vi "240913.vi"() -> ()   [LabVIEW 2024]
panel:
  in  "stop":bool
  in  "num":i8
  out "?":bool
  out "?":bool
  out "?":bool
  out "?":bool
  out "?":bool
  out "?":bool
  out "?":bool
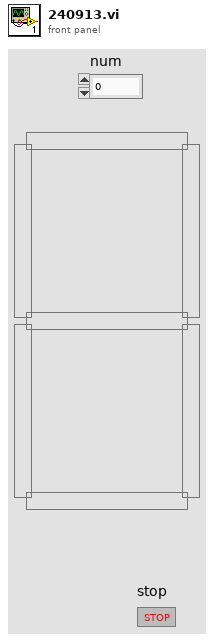
[diagram p1: front panel]
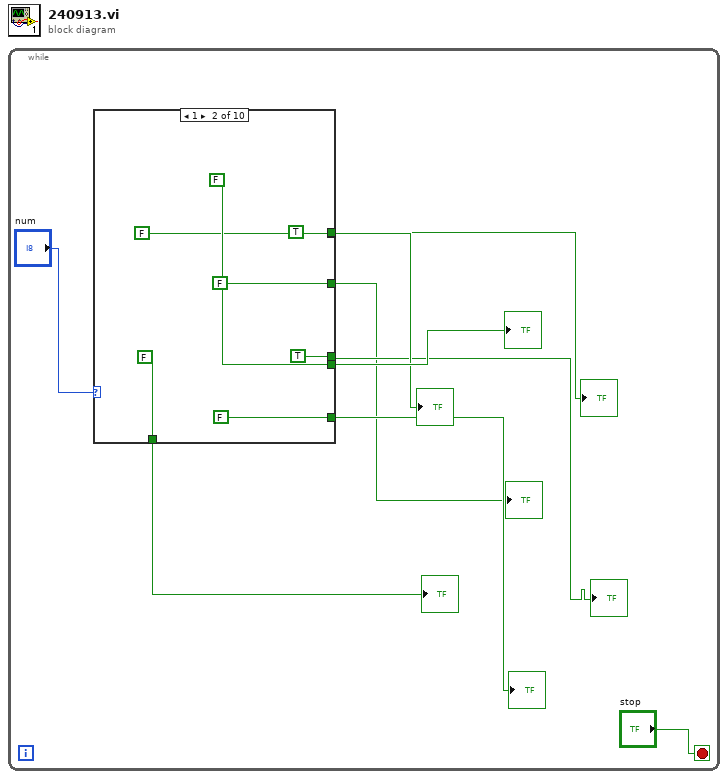
[diagram p0: block diagram]
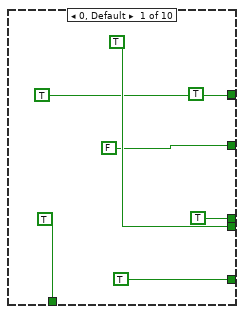
[diagram p2: hidden frame]
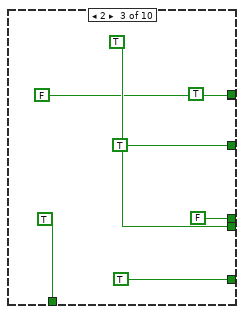
[diagram p3: hidden frame]
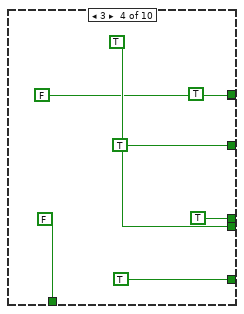
[diagram p4: hidden frame]
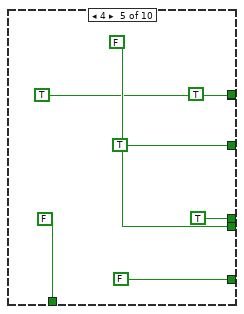
[diagram p5: hidden frame]
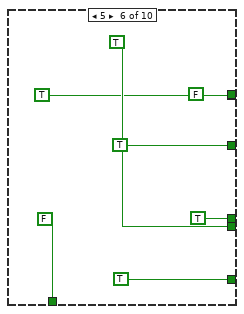
[diagram p6: hidden frame]
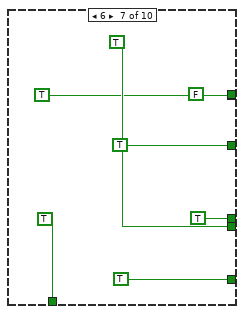
[diagram p7: hidden frame]
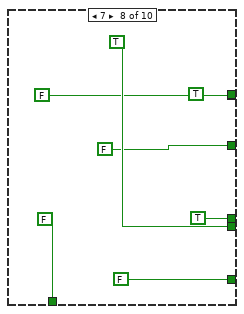
[diagram p8: hidden frame]
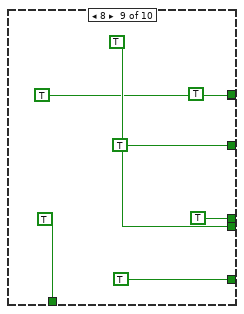
[diagram p9: hidden frame]
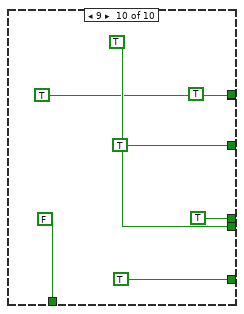
[diagram p10: hidden frame]
diagram:
  n1 = while {
    stop <- "stop" stop-if-true
    n2 = case shown="1" "num" {
      tunnel: [TRUE ("OK Button") FALSE ("OK Button") TRUE ("OK Button") TRUE ("OK Button") FALSE ("OK Button") TRUE ("OK Button") TRUE ("OK Button") TRUE ("OK Button") TRUE ("OK Button") TRUE ("OK Button")] -> w9
      tunnel: [TRUE ("OK Button") FALSE ("OK Button") FALSE ("OK Button") FALSE ("OK Button") TRUE ("OK Button") TRUE ("OK Button") TRUE ("OK Button") FALSE ("OK Button") TRUE ("OK Button") TRUE ("OK Button")] -> w8
      tunnel: [TRUE ("OK Button") FALSE ("OK Button") TRUE ("OK Button") FALSE ("OK Button") FALSE ("OK Button") FALSE ("OK Button") TRUE ("OK Button") FALSE ("OK Button") TRUE ("OK Button") FALSE ("OK Button")] -> w7
      tunnel: [TRUE ("OK Button") FALSE ("OK Button") TRUE ("OK Button") TRUE ("OK Button") FALSE ("OK Button") TRUE ("OK Button") TRUE ("OK Button") FALSE ("OK Button") TRUE ("OK Button") TRUE ("OK Button")] -> w6
      tunnel: [TRUE ("OK Button") TRUE ("OK Button") FALSE ("OK Button") TRUE ("OK Button") TRUE ("OK Button") TRUE ("OK Button") TRUE ("OK Button") TRUE ("OK Button") TRUE ("OK Button") TRUE ("OK Button")] -> w5
      tunnel: [FALSE ("OK Button") FALSE ("OK Button") TRUE ("OK Button") TRUE ("OK Button") TRUE ("OK Button") TRUE ("OK Button") TRUE ("OK Button") FALSE ("OK Button") TRUE ("OK Button") TRUE ("OK Button")] -> w4
      tunnel: [TRUE ("OK Button") TRUE ("OK Button") TRUE ("OK Button") TRUE ("OK Button") TRUE ("OK Button") FALSE ("OK Button") FALSE ("OK Button") TRUE ("OK Button") TRUE ("OK Button") TRUE ("OK Button")] -> w3
      frame 0, Default {
      }
      frame 1 {
      }
      frame 2 {
      }
      frame 3 {
      }
      frame 4 {
      }
      frame 5 {
      }
      frame 6 {
      }
      frame 7 {
      }
      frame 8 {
      }
      frame 9 {
      }
    }
    "?" <- w9
    "?" <- w6
    "?" <- w4
    "?" <- w3
    "?" <- w5
    "?" <- w7
    "?" <- w8
  }
